vi "SP Execute Test.vi"(1 "CH Controls":T13[](array[typedef]) {"Measure" items=["S11", "S21", "S12", "S22"]; "Reference" format="%#.2g"; "Display Data" items=["Data", "Memory", "Data/Memory"]; "Format" items=["Log Mag", "Phase", "Expanded Phase", "Delay", "Smith", "Polar", "Lin Mag", "SWR", "Loss", "Real", "Imaginary"]; "Scale" min=0.001 step=1.0 format="%#.2g"; "Position" min=0.0 max=10.0}, 5 "Seq Count":u32, 7 "Timing Metrics In":string, 9 "Test Parameters":T20={"Stimulus"={"Use Instrument Settings"=FALSE, "Blank Frequencies"=FALSE, "Sweep Type"=enum."Linear", "Sweep"={"Fstart"=500.0, "Fstop"=1500.0, "Units"=enum."MHz", "Points"=2}, "Power (dBm)"=999.0, "IFBW (Hz)"=-1.0, "Sweep Time (s)"=-1.0, "Calibration"={"State"=FALSE, "String"=""}}, "Measurement"={"Auto Select"=TRUE, "Data Source"=enum."VNA", "Ports"=2, "Parameters"=[]}, "De-Embed"={"De-Embed"=FALSE, "Adapters"=[]}, "Display"={"Lock Control"=FALSE, "Retain Settings"=TRUE, "Formatted Data"=FALSE, "Plot Orientation"=enum."Single", "Plot Controls"=[{"Trace Orientation"=enum."Overlay", "Frequency"={"Change Frequency"=FALSE, "Start"=500.0, "Stop"=1500.0, "Units"=enum."MHz"}, "Markers"=[], "Traces"=[]}, {"Trace Orientation"=enum."Overlay", "Frequency"={"Change Frequency"=FALSE, "Start"=500.0, "Stop"=1500.0, "Units"=enum."MHz"}, "Markers"=[], "Traces"=[]}, {"Trace Orientation"=enum."Overlay", "Frequency"={"Change Frequency"=FALSE, "Start"=500.0, "Stop"=1500.0, "Units"=enum."MHz"}, "Markers"=[], "Traces"=[]}, {"Trace Orientation"=enum."Overlay", "Frequency"={"Change Frequency"=FALSE, "Start"=500.0, "Stop"=1500.0, "Units"=enum."MHz"}, "Markers"=[], "Traces"=[]}]}, "Limits"=[], "Filter Limits"=[]} {"Filter Limits"."Parameter"."Stimulus Port" min=1 step=1; "Filter Limits"."Parameter"."Response Port" min=1 step=1; "Filter Limits"."Passband"."Bandwidth Attn" format="%.3g"; "Filter Limits"."Passband"."Stop/Span" format="%.3g"; "Filter Limits"."Passband"."Start/Center" format="%.3g"; "Measurement"."Parameters"."Channel" min=0 max=32 step=1; "Measurement"."Parameters"."Parameter"."Stimulus Port" min=1 step=1; "Measurement"."Parameters"."Parameter"."Response Port" min=1 step=1; "Limits"."Parameter"."Stimulus Port" min=1 step=1; "Limits"."Parameter"."Response Port" min=1 step=1; "Stimulus"."Sweep Time (s)" format="%.3g"; "Display"."Plot Controls"."Traces"."Reference" format="%#.2g"; "Display"."Plot Controls"."Traces"."Display Data" items=["Data", "Memory", "Data/Memory"]; "Display"."Plot Controls"."Traces"."Format" items=["Log Mag", "Phase", "Expanded Phase", "Delay", "Smith", "Polar", "Lin Mag", "SWR", "Loss", "Real", "Imaginary"]; "Display"."Plot Controls"."Traces"."Scale" min=0.001 step=1.0 format="%#.2g"; "Display"."Plot Controls"."Traces"."Position" min=0.0 max=10.0; "Display"."Plot Controls"."Frequency"."Stop" format="%.3g"; "Display"."Plot Controls"."Frequency"."Start" format="%.3g"}, 11 "error in (no error)":errorcluster, 12 "Driver Refs":T16, 13 "Instrument Record":T9) -> (3 "Limit Results":T1[](array[typedef]) {"Parameter"."Stimulus Port" min=1 step=1; "Parameter"."Response Port" min=1 step=1}, 4 "Results":waveform(dbl)[](array[waveform]), 6 "Memory Exists?":bool[](array[boolean]), 8 "Timing Metrics Out":string, 10 "Parameters Measured":T10[](array[typedef]) {"Channel" min=1 max=99 step=1; "Parameter"."Stimulus Port" min=1 step=1; "Parameter"."Response Port" min=1 step=1}, 14 "Passed?":bool, 15 "error out":errorcluster)   [LabVIEW 2011]
uses:
  TypeDefs/SP Test Parameters.ctl
  TypeDefs/SP Stimulus Parameters.ctl
  TypeDefs/SP Frequency Units.ctl
  TypeDefs/SP Calibration State.ctl
  TypeDefs/SP Measurement.ctl
  TypeDefs/SP Parameters.ctl
  TypeDefs/SP Parameter.ctl
  TypeDefs/SP De-Embed.ctl
  TypeDefs/SP Adapter.ctl
  TypeDefs/SP Data.ctl
  TypeDefs/SP Display Parameters.ctl
  TypeDefs/SP Display Plot Controls Cluster.ctl
  TypeDefs/SP Marker Cluster.ctl
  TypeDefs/SP Marker Type.ctl
  TypeDefs/SP Display Trace Controls.ctl
  TypeDefs/SP Display Format.ctl
  TypeDefs/SP Display Data.ctl
  TypeDefs/SP Limit.ctl
  TypeDefs/SP Format.ctl
  TypeDefs/SP Limit Type.ctl
  TypeDefs/SP Limit Point.ctl
  Test Referential Limit.ctl
  TypeDefs/SP Filter.ctl
  TypeDefs/SP Filter Type.ctl
  TypeDefs/SP Filter Passband.ctl
  TypeDefs/SP Frequency Format.ctl
  TypeDefs/SP Filter Ripple.ctl
  TypeDefs/SP Attenuation Point.ctl
  TypeDefs/SP Attenuation Type.ctl
  TypeDefs/SP Skirt Rejection Point.ctl
  TypeDefs/SP Relative Loss.ctl
  TypeDefs/SP Driver Refs.ctl
  drivers/VNA/VNA Driver Ref.ctl
  drivers/SNA/SNA Driver Ref.ctl
  drivers/IMP/IMP Driver Ref.ctl
  TypeDefs/SP Parameter to Measure.ctl
  TypeDefs/SP Measurement Format.ctl
  typedefs/Instrument Record.ctl
  TypeDefs/SP Limit Results.ctl
  TypeDefs/SP Bandwidth Limit Results.ctl
  TypeDefs/SP Ripple Limit Results.ctl
  TypeDefs/SP Attenuation Limit Results.ctl
  TypeDefs/SP Skirt Limit Results.ctl
  TypeDefs/SP Miscellaneous Parameters.ctl
  drivers/VNA/VNA Command.ctl
  drivers/SNA/SNA Command.ctl
  drivers/IMP/S2P/TypeDefs/S2P IMP Measurement Data.ctl
  drivers/IMP/IMP Command.ctl
panel:
  in  "Empty Results":waveform(dbl)[](array[waveform])
  # "Div"
  # "Div"
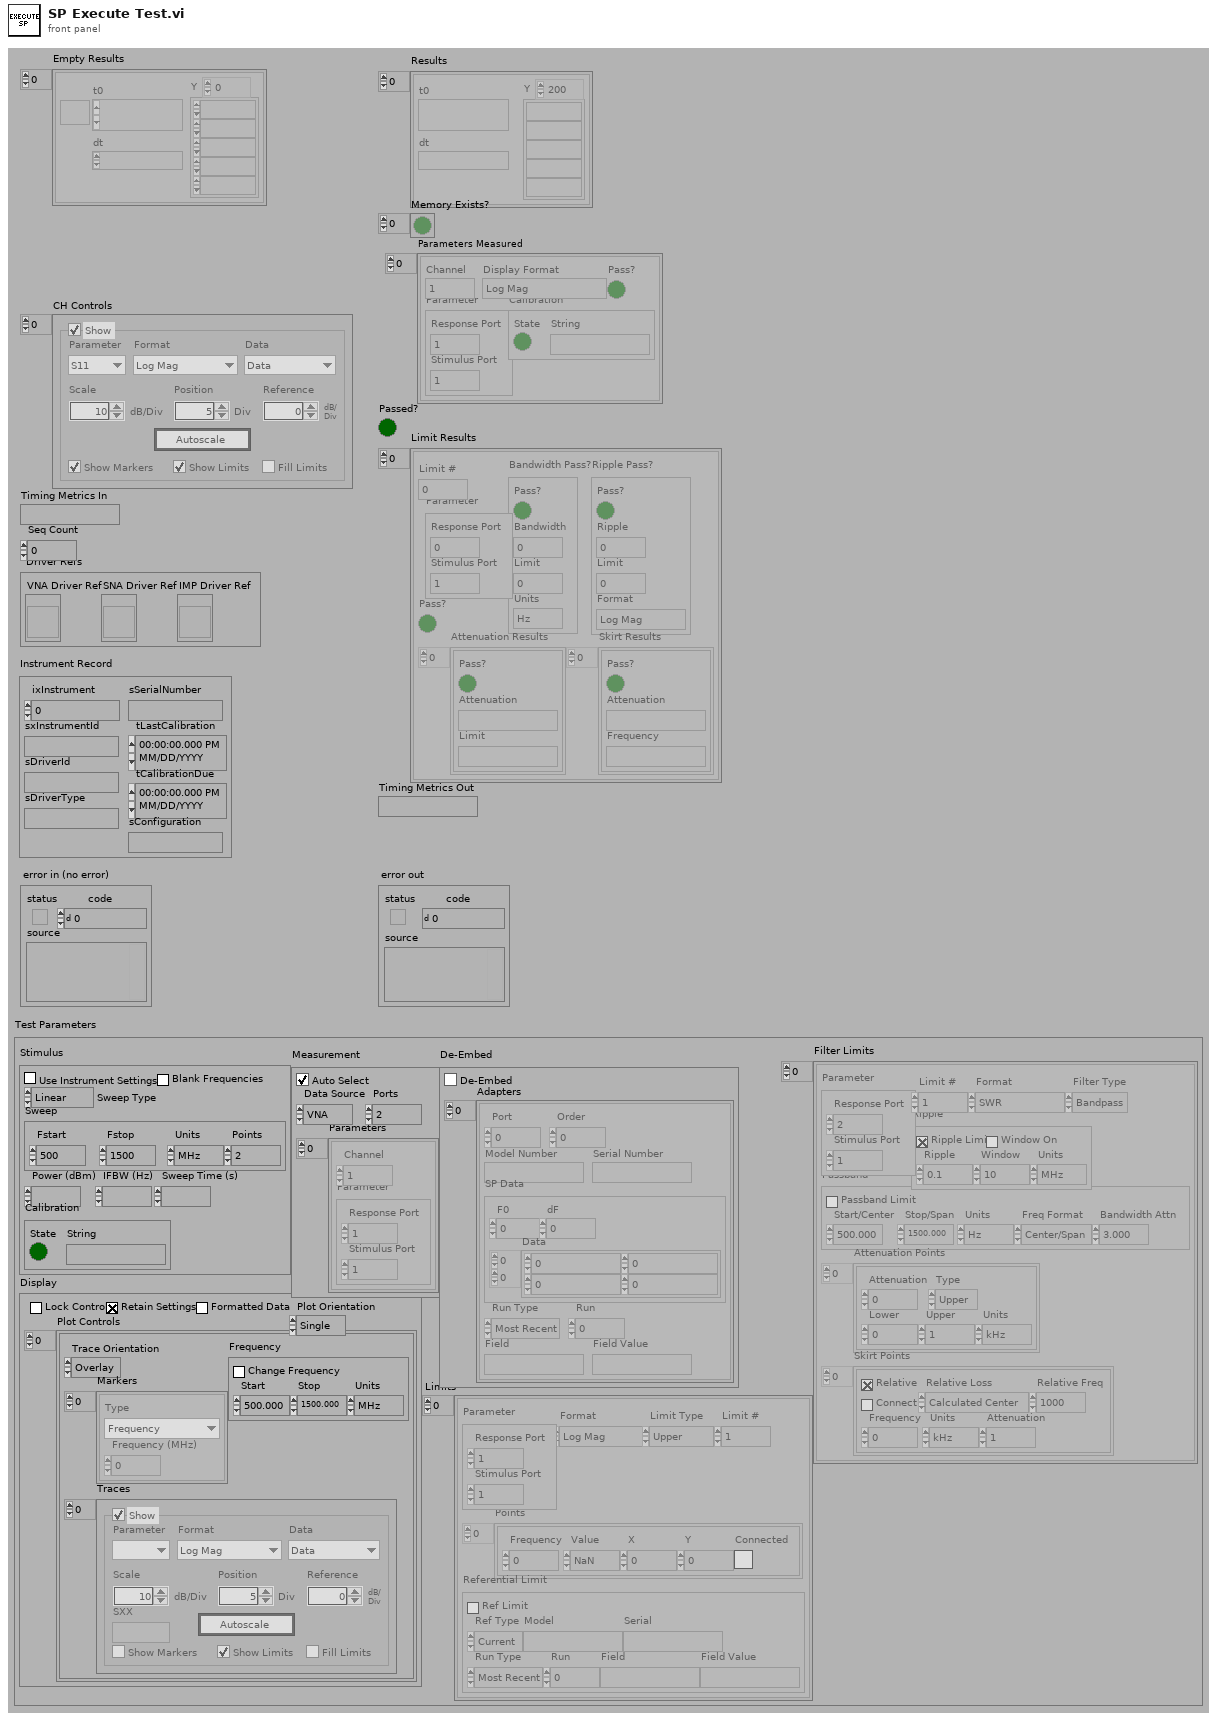
[diagram p1: front panel]
types:
  T1 = typedef "SP Limit Results.ctl" = cluster{"Limit #":i8, "Parameter":T2, "Bandwidth Pass?":T3, "Ripple Pass?":T5, "Attenuation Results":T7[], "Skirt Results":T8[], "Pass?":bool}
  T2 = typedef "SP Parameter.ctl" = cluster{"Stimulus Port":i8, "Response Port":i8}
  T3 = typedef "SP Bandwidth Limit Results.ctl" = cluster{"Pass?":bool, "Bandwidth":dbl, "Limit":dbl, "Units":T4}
  T4 = typedef "SP Frequency Units.ctl" = enum16{"Hz", "kHz", "MHz", "GHz", "Points"}
  T5 = typedef "SP Ripple Limit Results.ctl" = cluster{"Pass?":bool, "Ripple":dbl, "Limit":dbl, "Format":T6}
  T6 = typedef "SP Format.ctl" = enum16{"Log Mag", "Lin Mag", "SWR", "Phase", "Expanded Phase", "Delay", "Insertion Loss", "Isolation", "Return Loss"}
  T7 = typedef "SP Attenuation Limit Results.ctl" = cluster{"Pass?":bool, "Attenuation":string, "Limit":string}
  T8 = typedef "SP Skirt Limit Results.ctl" = cluster{"Pass?":bool, "Attenuation":string, "Frequency":string}
  T9 = typedef "Instrument Record.ctl" = cluster{"ixInstrument":i32, "sxInstrumentId":string, "sDriverId":string, "sDriverType":string, "sSerialNumber":string, "tLastCalibration":timestamp, "tCalibrationDue":timestamp, "sConfiguration":string}
  T10 = typedef "SP Parameter to Measure.ctl" = cluster{"Channel":i8, "Parameter":T2, "Calibration":T11, "Display Format":T12, "Pass?":bool}
  T11 = typedef "SP Calibration State.ctl" = cluster{"State":bool, "String":string}
  T12 = typedef "SP Measurement Format.ctl" = enum32{"Log Mag", "Phase", "Delay", "Smith (R+jX)", "Polar (Re/Im)", "Linear Mag", "SWR", "Real", "Imaginary", "Smith (Lin/Phase)", "Smith (Log/Phase)", "Smith (Real/Imag)", "Smith (G+jB)", "Polar (Lin/Phase)", "Polar (Log/Phase)", "Expanded Phase", "Positive Phase", "Inverted Smith", "Unwrapped Phase", "Power Out", "Power In", "Linear Mag/Phase", "Log Mag/Phase", "Real/Imaginary"}
  T13 = typedef "SP Display Trace Controls.ctl" = cluster{"Trace On":bool, "Measure":i32, "Format":T14, "Autoscale":bool, "Reference":dbl, "\nRefUnit":string, "Position":dbl, "Scale":dbl, "ScaleUnit":string, "LimitOn":bool, "LimitFill":bool, "Display Data":T15, "Show Markers":bool, "SXX":string}
  T14 = typedef "SP Display Format.ctl" = i32
  T15 = typedef "SP Display Data.ctl" = u16
  T16 = typedef "SP Driver Refs.ctl" = cluster{"VNA Driver Ref":T17, "SNA Driver Ref":T18, "IMP Driver Ref":T19}
  T17 = typedef "VNA Driver Ref.ctl" = refnum<vi>
  T18 = typedef "SNA Driver Ref.ctl" = refnum<vi>
  T19 = typedef "IMP Driver Ref.ctl" = refnum<vi>
  T20 = typedef "SP Test Parameters.ctl" = cluster{"Stimulus":T21, "Measurement":T22, "De-Embed":T24, "Display":T27, "Limits":T31[], "Filter Limits":T35[]}
  T21 = typedef "SP Stimulus Parameters.ctl" = cluster{"Use Instrument Settings":bool, "Blank Frequencies":bool, "Sweep Type":enum32{"Linear", "Logarithmic", "List", "Power", "CW"}, "Sweep":cluster{"Fstart":dbl, "Fstop":dbl, "Units":T4, "Points":i32}, "Power (dBm)":dbl, "IFBW (Hz)":dbl, "Sweep Time (s)":dbl, "Calibration":T11}
  T22 = typedef "SP Measurement.ctl" = cluster{"Auto Select":bool, "Data Source":enum16{"VNA", "Data File"}, "Ports":i8, "Parameters":T23[]}
  T23 = typedef "SP Parameters.ctl" = cluster{"Channel":i8, "Parameter":T2}
  T24 = typedef "SP De-Embed.ctl" = cluster{"De-Embed":bool, "Adapters":T25[]}
  T25 = typedef "SP Adapter.ctl" = cluster{"Port":i8, "Order":i8, "Model Number":string, "Serial Number":string, "SP Data":T26, "Run Type":enum16{"Most Recent", "Run #", "Match Field"}, "Run":i32, "Field":string, "Field Value":string}
  T26 = typedef "SP Data.ctl" = cluster{"F0":dbl, "dF":dbl, "Data":cdb[][]}
  T27 = typedef "SP Display Parameters.ctl" = cluster{"Lock Control":bool, "Retain Settings":bool, "Formatted Data":bool, "Plot Orientation":enum32{"Single", "Dual", "Quad"}, "Plot Controls":T28[]}
  T28 = typedef "SP Display Plot Controls Cluster.ctl" = cluster{"Trace Orientation":enum32{"Overlay", "Split"}, "Frequency":cluster{"Change Frequency":bool, "Start":dbl, "Stop":dbl, "Units":T4}, "Markers":T29[], "Traces":T13[]}
  T29 = typedef "SP Marker Cluster.ctl" = cluster{"Type":T30, "Frequency (MHz)":dbl}
  T30 = typedef "SP Marker Type.ctl" = enum16{"Frequency", "Trace Maximum", "Trace Minimum", "Limit Maximum", "Limit Minimum"}
  T31 = typedef "SP Limit.ctl" = cluster{"Parameter":T2, "Format":T6, "Limit Type":T32, "Points":T33[], "Referential Limit":T34, "Limit #":i8}
  T32 = typedef "SP Limit Type.ctl" = enum16{"Upper", "Lower", "Delta", "Filter", "Referential"}
  T33 = typedef "SP Limit Point.ctl" = cluster{"Frequency":dbl, "Value":dbl, "X":dbl, "Y":dbl, "Connected":bool}
  T34 = typedef "Test Referential Limit.ctl" = cluster{"Ref Limit":bool, "Ref Type":enum16{"Current", "Specify"}, "Model":string, "Serial":string, "Run Type":enum16{"Most Recent", "Run #", "Match Field"}, "Run":i32, "Field":string, "Field Value":string}
  T35 = typedef "SP Filter.ctl" = cluster{"Limit #":i8, "Parameter":T2, "Format":T6, "Filter Type":T36, "Passband":T37, "Ripple":T39, "Attenuation Points":T40[], "Skirt Points":T42[]}
  T36 = typedef "SP Filter Type.ctl" = enum16{"Lowpass", "Highpass", "Bandpass", "Bandstop"}
  T37 = typedef "SP Filter Passband.ctl" = cluster{"Start/Center":dbl, "Stop/Span":dbl, "Units":T4, "Freq Format":T38, "Bandwidth Attn":dbl, "Passband Limit":bool}
  T38 = typedef "SP Frequency Format.ctl" = enum16{"Start/Stop", "Center/Span"}
  T39 = typedef "SP Filter Ripple.ctl" = cluster{"Ripple Limit":bool, "Window On":bool, "Ripple":dbl, "Window":dbl, "Units":T4}
  T40 = typedef "SP Attenuation Point.ctl" = cluster{"Attenuation":dbl, "Type":T41, "Lower":dbl, "Upper":dbl, "Units":T4}
  T41 = typedef "SP Attenuation Type.ctl" = enum16{"Center", "Lower", "Upper"}
  T42 = typedef "SP Skirt Rejection Point.ctl" = cluster{"Relative":bool, "Connect":bool, "Frequency":dbl, "Units":T4, "Attenuation":dbl, "Relative Loss":T43, "Relative Freq":dbl}
  T43 = typedef "SP Relative Loss.ctl" = enum16{"Calculated Center", "Passband Minimum", "Passband Maximum", "Passband Average", "Frequency"}
  T44 = cluster{"Measurement Units":T4, "Display Units":T4}
  T45 = typedef "SP Miscellaneous Parameters.ctl" = cluster{"Formatted Data":bool, "Auto Select":bool, "Seq Count":u32}
  T46 = typedef "VNA Command.ctl" = enum16{"LOAD", "INITIALIZE", "PRESET", "GET STIMULUS", "SET STIMULUS", "GET CALIBRATION", "CALIBRATE", "RESTORE", "MEASURE", "RELEASE", "UNLOAD", "CONFIRM", "SORT"}
  T47 = typedef "SNA Command.ctl" = enum16{"LOAD", "INITIALIZE", "PRESET", "GET STIMULUS", "SET STIMULUS", "GET CALIBRATION", "CALIBRATE", "RESTORE", "MEASURE", "RELEASE", "UNLOAD", "CONFIRM", "SORT"}
  T48 = typedef "S2P IMP Measurement Data.ctl" = cluster{"Parameters Measured":T10[], "S2P Data":T26}
  T49 = typedef "IMP Command.ctl" = enum16{"LOAD", "INITIALIZE", "IMPORT", "UNLOAD"}
  T50 = cluster{"F0":dbl, "dF":dbl, "Formatted Values":dbl[]}
  T51 = cluster{"Bandwidth Attn":dbl, "Center Freq (MHz)":dbl, "Span Freq (MHz)":dbl, "Pass?":bool, "Bandwidth (MHz)":dbl, "Bandwidth Limit (MHz)":dbl, "Attenuation Points":dbl[]}
  T52 = cluster{"Upper Limit":cluster{"F0":dbl, "dF":dbl, "Formatted Values":dbl[]}, "Lower Limit":cluster{"F0":dbl, "dF":dbl, "Formatted Values":dbl[]}}
  T53 = cluster{"UPass?":bool, "LPass?":bool, "Frequency":dbl, "Lower Limit":dbl, "Upper Limit":dbl, "Type":T41}[]
  T54 = cluster{"x0":dbl, "dx":dbl, "Stored Values":dbl[]}
  T55 = cluster{cluster{"x0":dbl, "dx":dbl, "Stored Values":dbl[]}, cluster{"x0":dbl, "dx":dbl, "Stored Values":dbl[]}}
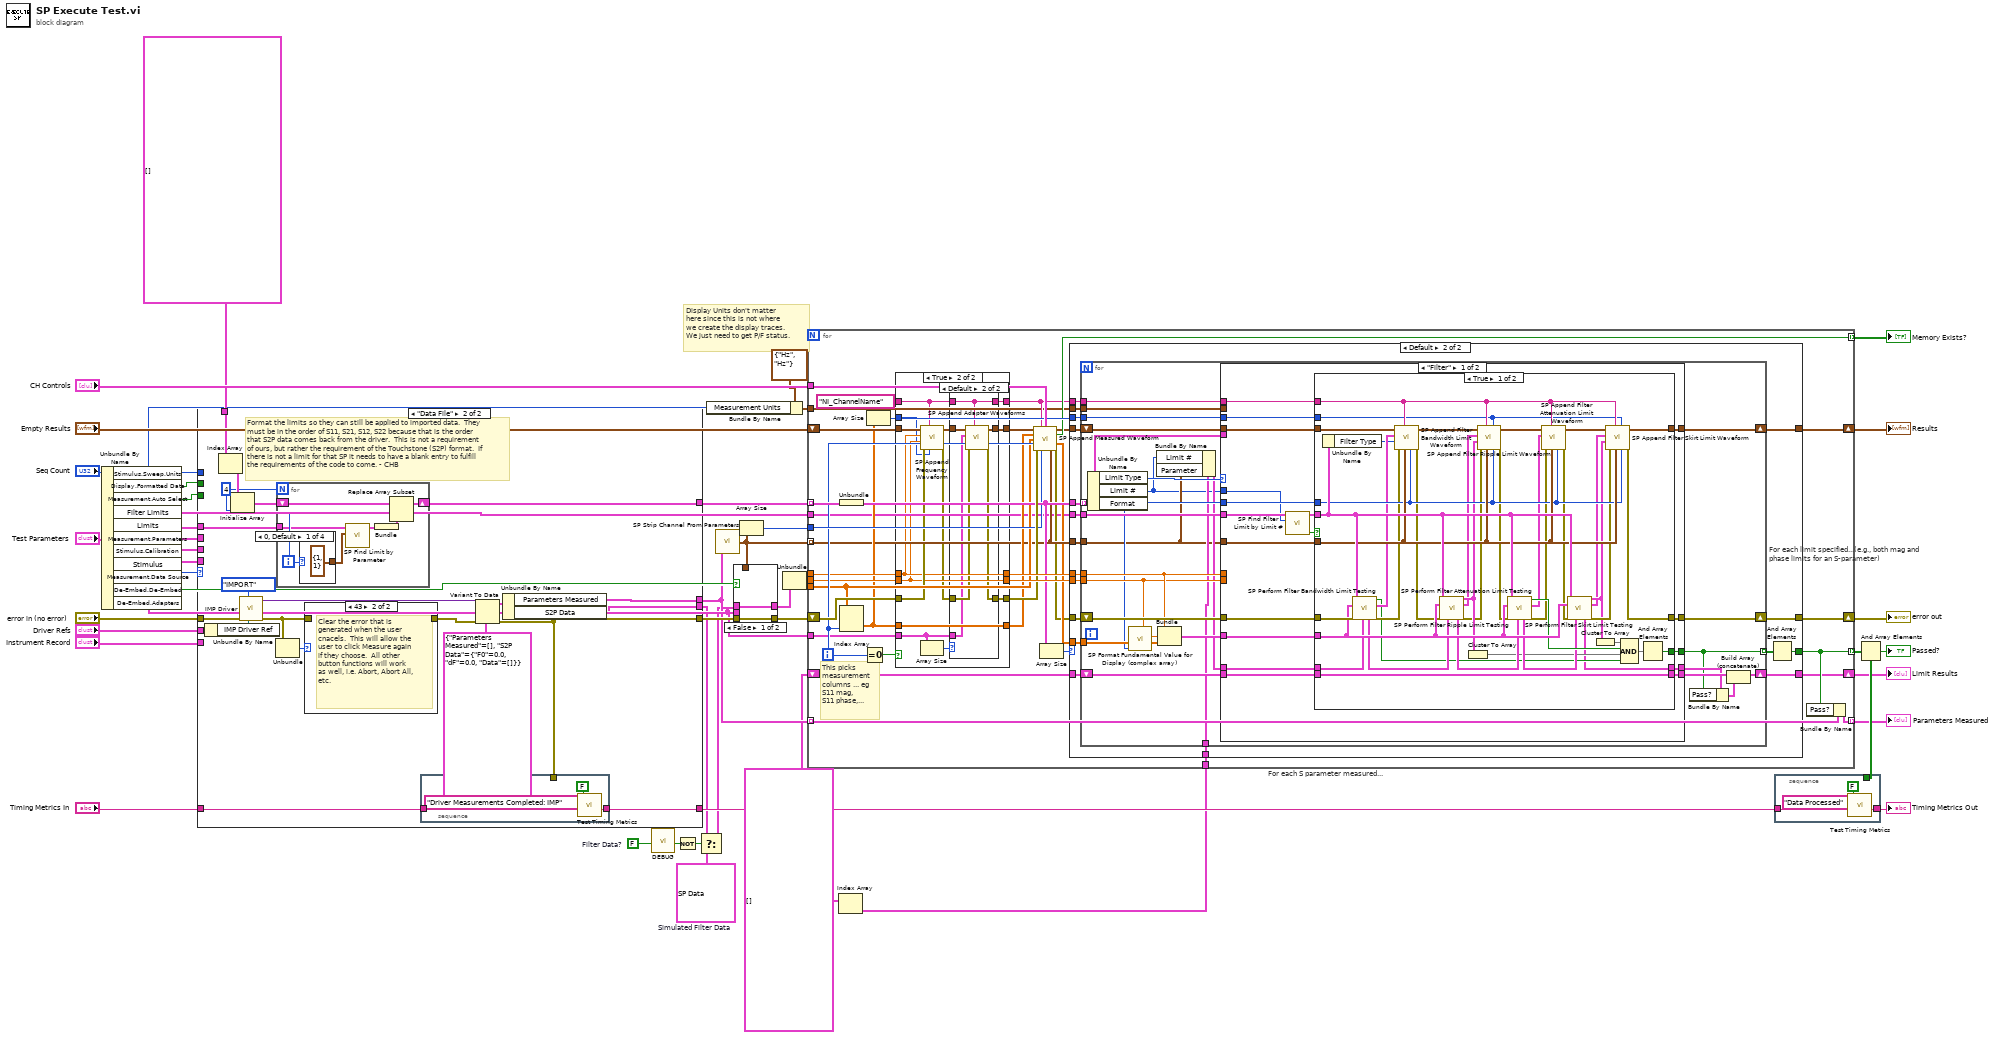
[diagram p0: block diagram]
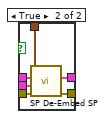
[diagram p2: hidden frame]
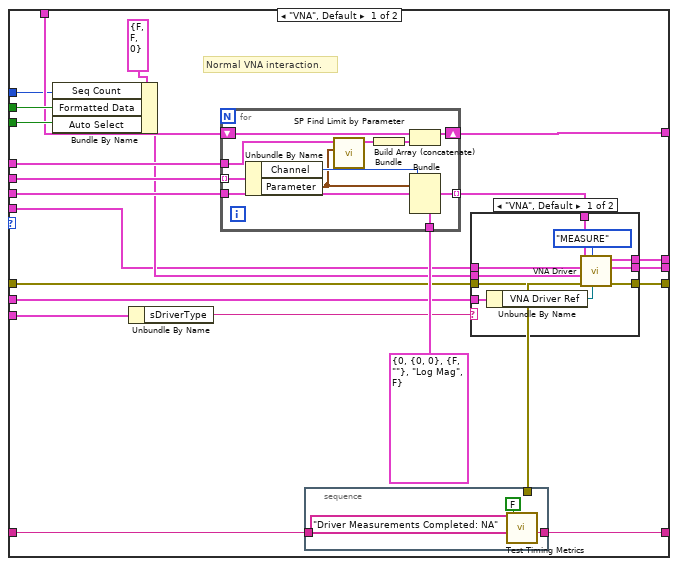
[diagram p3: hidden frame]
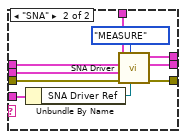
[diagram p4: hidden frame]
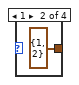
[diagram p6: hidden frame]
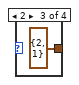
[diagram p7: hidden frame]
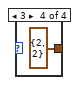
[diagram p8: hidden frame]
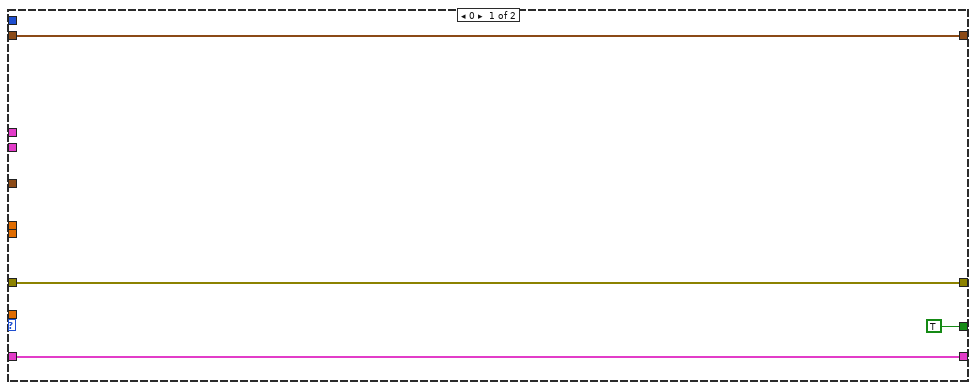
[diagram p9: hidden frame]
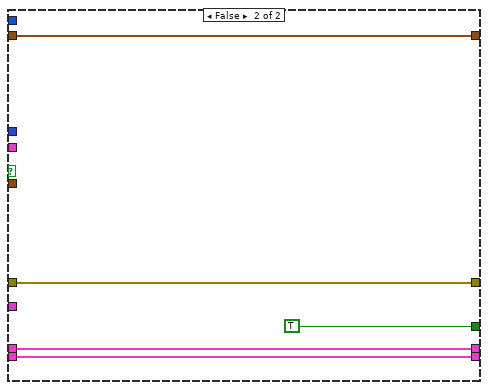
[diagram p10: hidden frame]
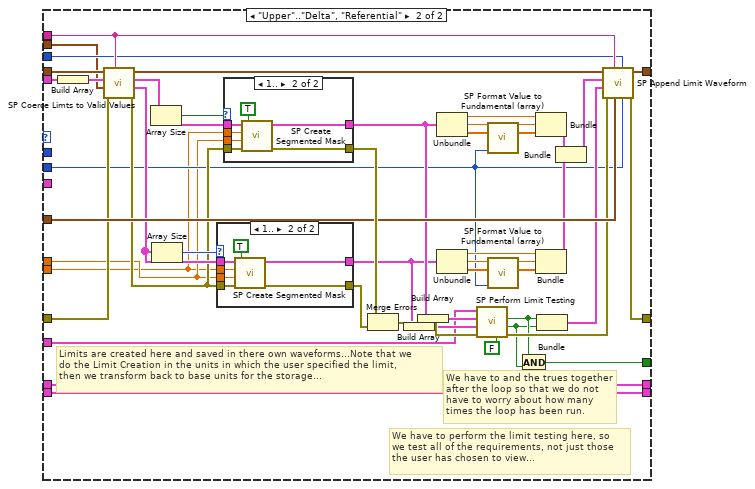
[diagram p11: hidden frame]
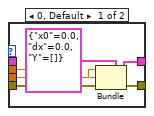
[diagram p12: hidden frame]
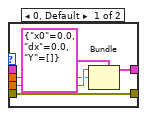
[diagram p13: hidden frame]
diagram:
  w3 = T1[] []
  w9 = FALSE  # Filter Data?
  w6 = T26 {"F0"=1700.0, "dF"=1.0, "Data"=[[-0.6018883288138366-0.2912013889246391i, 0.25843199895687796+0.6001894532665946i, 1.0+0.0i, 1.0+0.0i], [-0.5763938433657362-0.16773283578975615i, 0.37772558398449546+0.6071698116448432i, 1.0+0.0i, 1.0+0.0i], [-0.519689947876343-0.05406961123928598i, 0.5054119893123452+0.5838015468749106i, 1.0+0.0i, 1.0+0.0i], [-0.4366631932536643+0.038653140967053336i, 0.6323001346464633+0.5273763672849814i, 1.0+0.0i, 1.0+0.0i], [-0.3367762107137387+0.10167424321959725i, 0.7461057345374577+0.4390505932852546i, 1.0+0.0i, 1.0+0.0i], [-0.23206146469338626+0.1317558747901435i, 0.8374292632292502+0.3249695878798761i, 1.0+0.0i, 1.0+0.0i], [-0.13428970687981837+0.1316706711180515i, 0.900317905750139+0.1948071131291862i, 1.0+0.0i, 1.0+0.0i], [-0.0519954009317567+0.10798684987828776i, 0.9338709717280576+0.05829020485907047i, 1.0+0.0i, 1.0+0.0i], [0.010578915376855002+0.06919151060092682i, 0.9411153215780537-0.07694445704762284i, 1.0+0.0i, 1.0+0.0i], [0.05258172168640398+0.02288386508379801i, 0.9247525186312551-0.20416450691947172i, 1.0+0.0i, 1.0+0.0i], [0.07586320408971295-0.02427093912251751i, 0.8912400676746711-0.3217436008032638i, 1.0+0.0i, 1.0+0.0i], [0.0834246197482034-0.06790328480338377i, 0.8439917666780876-0.42831686461220936i, 1.0+0.0i, 1.0+0.0i], [0.07866808071336005-0.10505806260292615i, 0.78641056187367-0.5234791187831817i, 1.0+0.0i, 1.0+0.0i], [0.06489162284893765-0.13445634684056035i, 0.7212501289028754-0.6083145624168425i, 1.0+0.0i, 1.0+0.0i], [0.04507227165494071-0.15522420928026068i, 0.6495134688280773-0.6824883986293371i, 1.0+0.0i, 1.0+0.0i], [0.02186237509833218-0.16744628811960777i, 0.5727083373218407-0.7463211066382691i, 1.0+0.0i, 1.0+0.0i], [-0.0028246619373131676-0.17163375094123137i, 0.4918939724054302-0.8016715915329948i, 1.0+0.0i, 1.0+0.0i], [-0.02714462258660534-0.16846044251443718i, 0.40771953951852236-0.848048518977557i, 1.0+0.0i, 1.0+0.0i], [-0.04965487991424324-0.15891144281898575i, 0.32087934927959744-0.8851169409466159i, 1.0+0.0i, 1.0+0.0i], [-0.06940115989214148-0.14395347580736373i, 0.23105911621068337-0.9151527346496748i, 1.0+0.0i, 1.0+0.0i], [-0.08515954507306635-0.12468116376469908i, 0.1403489417912114-0.9346160952374049i, 1.0+0.0i, 1.0+0.0i], [-0.09674321476559439-0.1023120232228757i, 0.04818766902243024-0.9456399069017796i, 1.0+0.0i, 1.0+0.0i], [-0.10384848778239429-0.07792886127276757i, -0.044093597115198176-0.9476633622454788i, 1.0+0.0i, 1.0+0.0i], [-0.10642398257790069-0.052629906048574614i, -0.13557150924760691-0.9402477642662153i, 1.0+0.0i, 1.0+0.0i], [-0.10447933019033262-0.027496582837167702i, -0.22651251036758296-0.9249390180549153i, 1.0+0.0i, 1.0+0.0i], [-0.09846522597296979-0.0033023854612930694i, -0.3150646229058073-0.9007516295430944i, 1.0+0.0i, 1.0+0.0i], [-0.08867113842250143+0.018985327208484115i, -0.3996975613559442-0.867381307278978i, 1.0+0.0i, 1.0+0.0i], [-0.07586177040152732+0.03886020162270151i, -0.4809323563603943-0.8261918442002553i, 1.0+0.0i, 1.0+0.0i], [-0.06076646059838993+0.055993218767238i, -0.5581660126308761-0.7778153443708942i, 1.0+0.0i, 1.0+0.0i], [-0.04381207606238176+0.06982104609066907i, -0.6287295195292726-0.7219563939864023i, 1.0+0.0i, 1.0+0.0i], [-0.02591401637984273+0.08040210957536097i, -0.6940277277339839-0.6599926809567306i, 1.0+0.0i, 1.0+0.0i], [-0.007662933312265582+0.08775248303207699i, -0.7520150911557977-0.5921261482908812i, 1.0+0.0i, 1.0+0.0i], [0.010327353173893283+0.09204591847645842i, -0.8054632379209045-0.5195334217200286i, 1.0+0.0i, 1.0+0.0i], [0.027570187893991904+0.09328646897248352i, -0.8495372541500987-0.4423692583583411i, 1.0+0.0i, 1.0+0.0i], [0.043636518509812976+0.09203190924415088i, -0.8866024628267639-0.3616497030468273i, 1.0+0.0i, 1.0+0.0i], [0.05815857292883628+0.08853217374133557i, -0.916102803615982-0.2779561134304512i, 1.0+0.0i, 1.0+0.0i], [0.07092777290362523+0.08316021939919031i, -0.9371691434087805-0.19228967425838717i, 1.0+0.0i, 1.0+0.0i], [0.08166451250945678+0.07633417924416686i, -0.9513886911911866-0.10464605910605339i, 1.0+0.0i, 1.0+0.0i], [0.09032871637381922+0.06840197558392054i, -0.956826030767709-0.016280501409187128i, 1.0+0.0i, 1.0+0.0i], [0.09705657838026943+0.05972833435455881i, -0.9541463163875222+0.07225510514550987i, 1.0+0.0i, 1.0+0.0i], [0.1017157657878945+0.05065605850842947i, -0.9433210671957775+0.16034009806172234i, 1.0+0.0i, 1.0+0.0i], [0.10448012976900736+0.041427625084476484i, -0.9245071206581749+0.2471693341448325i, 1.0+0.0i, 1.0+0.0i], [0.10542608402879289+0.032428786673877275i, -0.8975198220345031+0.33217007008156507i, 1.0+0.0i, 1.0+0.0i], [0.10466470261736624+0.02365108018246849i, -0.8626567303162795+0.414682914555206i, 1.0+0.0i, 1.0+0.0i], [0.10230330280167362+0.015328926437470256i, -0.8200935976978028+0.4940875957110222i, 1.0+0.0i, 1.0+0.0i], [0.09860433016372575+0.007612820033679798i, -0.7699420524716706+0.5693633026244502i, 1.0+0.0i, 1.0+0.0i], [0.09368580974287007+0.0005573491927782479i, -0.7125436571337076+0.6399868897098582i, 1.0+0.0i, 1.0+0.0i], [0.08756119563288138-0.005806518604850663i, -0.6484962392852844+0.7060130026305704i, 1.0+0.0i, 1.0+0.0i], [0.08041985909062076-0.011148728567773908i, -0.5775952397661317+0.7645606455570968i, 1.0+0.0i, 1.0+0.0i], [0.0721923675580467-0.01580110179377119i, -0.5008883448891464+0.8164731956480251i, 1.0+0.0i, 1.0+0.0i], [0.06304326080671951-0.019419514076621566i, -0.41869765614671717+0.8622852805854512i, 1.0+0.0i, 1.0+0.0i], [0.053113941666137324-0.02208180740934336i, -0.3318925693769244+0.8993924639844907i, 1.0+0.0i, 1.0+0.0i], [0.042327853302586-0.023652514838652564i, -0.24055892940082874+0.9288413877153515i, 1.0+0.0i, 1.0+0.0i], [0.030838926552563258-0.02377923837039422i, -0.1461630870200274+0.94816630091127i, 1.0+0.0i, 1.0+0.0i], [0.01870982273255544-0.02249094220644248i, -0.04987288285879495+0.9566115126117133i, 1.0+0.0i, 1.0+0.0i], [0.006143225202847295-0.019632915523019934i, 0.04882759736918653+0.9571527194865719i, 1.0+0.0i, 1.0+0.0i], [-0.006649233662454022-0.014947621089703395i, 0.14785104513947628+0.9464339527379307i, 1.0+0.0i, 1.0+0.0i], [-0.01940066611782043-0.008320788091237083i, 0.24621363044144073+0.9252244724465958i, 1.0+0.0i, 1.0+0.0i], [-0.031724477990716045+0.0004593234166332625i, 0.34334164002308953+0.8934780479138885i, 1.0+0.0i, 1.0+0.0i], [-0.04314760762766865+0.011362796606390155i, 0.4358039550543813+0.8497553136816223i, 1.0+0.0i, 1.0+0.0i], [-0.05318862373029016+0.024395123071694384i, 0.5259021789709166+0.7966200883485474i, 1.0+0.0i, 1.0+0.0i], [-0.06127106944236175+0.03943945567223453i, 0.6097426634187605+0.7326566320758651i, 1.0+0.0i, 1.0+0.0i], [-0.06679234071688708+0.05615716369606713i, 0.6867663672489616+0.6586197824203649i, 1.0+0.0i, 1.0+0.0i], [-0.0691744018739379+0.07405494542895746i, 0.7564985991167886+0.575499578950503i, 1.0+0.0i, 1.0+0.0i], [-0.06791698397038357+0.09252578356037992i, 0.8155353867263107+0.48347895828640297i, 1.0+0.0i, 1.0+0.0i], [-0.06252754216094453+0.11062154548610267i, 0.8642232625000523+0.3839108643796431i, 1.0+0.0i, 1.0+0.0i], [-0.05288141014773409+0.12739587954612072i, 0.9028158825599887+0.2775523651413829i, 1.0+0.0i, 1.0+0.0i], [-0.03894579332671778+0.14139470266136236i, 0.9280152441914633+0.16565062882775497i, 1.0+0.0i, 1.0+0.0i], [-0.021125341496806904+0.151477317248256i, 0.939894734553657+0.04956449848513996i, 1.0+0.0i, 1.0+0.0i], [-8.54153469215474e-05+0.15640582926585647i, 0.9376456681984923-0.06977512732062516i, 1.0+0.0i, 1.0+0.0i], [0.022929291642011577+0.15463846381715032i, 0.9199704468055506-0.19057784118682192i, 1.0+0.0i, 1.0+0.0i], [0.0464693495485323+0.14532227623577607i, 0.8863437141821184-0.31187044472783965i, 1.0+0.0i, 1.0+0.0i], [0.06796233423343687+0.12734375811660376i, 0.8345695367569668-0.4302649312109253i, 1.0+0.0i, 1.0+0.0i], [0.08500727751830782+0.10086621442731726i, 0.7647210645029121-0.5439587069427498i, 1.0+0.0i, 1.0+0.0i], [0.09449733566311004+0.06653208034100902i, 0.6762524317082488-0.6516719436743442i, 1.0+0.0i, 1.0+0.0i], [0.09329074668210832+0.026321785808147646i, 0.5677674949875572-0.7475681327174338i, 1.0+0.0i, 1.0+0.0i], [0.07865411994723565-0.016508336787470018i, 0.4400858149871239-0.8284769003283825i, 1.0+0.0i, 1.0+0.0i], [0.048803583668660194-0.0568001919793608i, 0.29465269320802007-0.8871734175171272i, 1.0+0.0i, 1.0+0.0i], [0.004182352171136945-0.08856370429529446i, 0.13510538282317108-0.9200123504592056i, 1.0+0.0i, 1.0+0.0i], [-0.05189515517396443-0.10516354963437015i, -0.03461173094638121-0.9233734570999651i, 1.0+0.0i, 1.0+0.0i], [-0.11271195420288169-0.10107101325115063i, -0.20690768709244398-0.8922502814371098i, 1.0+0.0i, 1.0+0.0i], [-0.16829804569833243-0.07347514401271295i, -0.3761310850654713-0.8257529634002132i, 1.0+0.0i, 1.0+0.0i], [-0.20548548055427257-0.024164447740455296i, -0.5338367606432877-0.7225856659800891i, 1.0+0.0i, 1.0+0.0i], [-0.21060051222683637+0.03808315595329911i, -0.6754503727190233-0.582206612212459i, 1.0+0.0i, 1.0+0.0i], [-0.17032472418299607+0.094645061065754i, -0.7947447285843722-0.3996471781744263i, 1.0+0.0i, 1.0+0.0i], [-0.07901238526411039+0.11140467318220737i, -0.8731045878321936-0.16488328715630465i, 1.0+0.0i, 1.0+0.0i], [0.041070055012981034+0.03384566989630328i, -0.8699933934683103+0.12689815077259753i, 1.0+0.0i, 1.0+0.0i], [0.09522272596441572-0.18030821997863317i, -0.7129285845384136+0.4292365673144433i, 1.0+0.0i, 1.0+0.0i], [-0.057767881783225034-0.44141158140544073i, -0.3949063232879774+0.5979367576916298i, 1.0+0.0i, 1.0+0.0i], [-0.38286646504616595-0.5339233635346229i, -0.08370031841862433+0.5428128260911925i, 1.0+0.0i, 1.0+0.0i], [-0.6707547787277324-0.419775731598612i, 0.07825384819214672+0.37890749400285856i, 1.0+0.0i, 1.0+0.0i], [-0.8355857960356216-0.22314755441846254i, 0.12261040144112519+0.2345446292020144i, 1.0+0.0i, 1.0+0.0i], [-0.9037567438213129-0.028112762066985517i, 0.11602268884490194+0.1383535085737117i, 1.0+0.0i, 1.0+0.0i], [-0.9169998461744372+0.13988503290590304i, 0.0949845629822241+0.08011970193404727i, 1.0+0.0i, 1.0+0.0i], [-0.899930373556771+0.27988017559060463i, 0.07315580096005365+0.045728264987258994i, 1.0+0.0i, 1.0+0.0i], [-0.8661043528407536+0.39413340338314434i, 0.054553862622702655+0.025635892912699222i, 1.0+0.0i, 1.0+0.0i], [-0.8243936793307876+0.48912918769055636i, 0.03991819386209603+0.013977392878197612i, 1.0+0.0i, 1.0+0.0i], [-0.7784470995137205+0.5678115679587512i, 0.028825584139034185+0.0072632962697511015i, 1.0+0.0i, 1.0+0.0i], [-0.7313802800212125+0.6348899971679764i, 0.0205487395382581+0.003472387393030255i, 1.0+0.0i, 1.0+0.0i], [-0.6837688567671468+0.6918431623911119i, 0.014419840627457749+0.0014134892277889925i, 1.0+0.0i, 1.0+0.0i], [-0.6365134789438374+0.7389840725178888i, 0.009920944480821309+0.0003505747060961784i, 1.0+0.0i, 1.0+0.0i], [-0.5904763409864403+0.7796262634874056i, 0.006653837313751247-0.00011408053981226363i, 1.0+0.0i, 1.0+0.0i], [-0.5458038211957541+0.8138547282240669i, 0.004300523219497427-0.0002554306678072595i, 1.0+0.0i, 1.0+0.0i], [-0.5022644767687758+0.8443413526481423i, 0.0026253146522399397-0.00022918787711075504i, 1.0+0.0i, 1.0+0.0i], [-0.46063758969998697+0.870834484803912i, 0.001436091657660389-0.00012640370942258324i, 1.0+0.0i, 1.0+0.0i], [-0.4205212715176568+0.892056364965568i, 0.0006149818521453536+8.922068080420638e-06i, 1.0+0.0i, 1.0+0.0i], [-0.38157455147732555+0.9109817304805171i, 5.375518211271426e-05+0.00014240657180357867i, 1.0+0.0i, 1.0+0.0i], [-0.34485224565543604+0.9272549765683717i, -0.00030340377232163763+0.0002531608231524423i, 1.0+0.0i, 1.0+0.0i], [-0.309191519645884+0.9410922014349631i, -0.0005289154873562566+0.00034528784815929107i, 1.0+0.0i, 1.0+0.0i], [-0.27508884312629384+0.9529178397253227i, -0.0006338801843677425+0.00040466816161339894i, 1.0+0.0i, 1.0+0.0i], [-0.2422478680394226+0.9628926910109905i, -0.0006939871891300646+0.0004435554302594064i, 1.0+0.0i, 1.0+0.0i], [-0.21065570740800724+0.9713087070604108i, -0.0006949515854707573+0.00046688773728251464i, 1.0+0.0i, 1.0+0.0i], [-0.18035111079641905+0.9790944797425006i, -0.0006601754880812151+0.0004626549083955471i, 1.0+0.0i, 1.0+0.0i], [-0.15169164023575432+0.9843406039366385i, -0.0006093961095685952+0.0004535171636329728i, 1.0+0.0i, 1.0+0.0i], [-0.12372146793299463+0.9890405004689183i, -0.0005414837854990509+0.0004127167055461758i, 1.0+0.0i, 1.0+0.0i], [-0.09768245673341534+0.992354807438694i, -0.00047695038839787676+0.000376764639465228i, 1.0+0.0i, 1.0+0.0i], [-0.07113158541444688+0.9955308991485885i, -0.0004038033811464111+0.0003282452010286005i, 1.0+0.0i, 1.0+0.0i], [-0.04617189233186482+0.9984217287640034i, -0.0003280045495189821+0.0002832338432393144i, 1.0+0.0i, 1.0+0.0i], [-0.022718715629611558+0.9993491168638301i, -0.0002576920416455954+0.00022080872682340007i, 1.0+0.0i, 1.0+0.0i], [9.899373129130176e-05+1.0003391503941879i, -0.00018868362455628517+0.0001505864199428088i, 1.0+0.0i, 1.0+0.0i], [0.021667480546618104+1.000266789369622i, -0.00013059902088087365+0.0001035530813307493i, 1.0+0.0i, 1.0+0.0i], [0.0436607778564319+1.0001804866206725i, -8.735516738020677e-05+3.889576665191044e-05i, 1.0+0.0i, 1.0+0.0i], [0.06449697829003033+1.000408654667916i, -3.166249611321768e-05-1.3981660909205915e-05i, 1.0+0.0i, 1.0+0.0i], [0.08391317799483462+0.998837524628444i, 2.4538463509062388e-05-7.002277693063898e-05i, 1.0+0.0i, 1.0+0.0i], [0.10290015988334145+0.9975167601003165i, 5.1350063085285844e-05-0.000112558866692047i, 1.0+0.0i, 1.0+0.0i], [0.120539997651031+0.9956299125744695i, 9.4619136097124e-05-0.000173838122966134i, 1.0+0.0i, 1.0+0.0i], [0.13920193906813186+0.9941959892829693i, 0.0001203264762262389-0.00022050148696545479i, 1.0+0.0i, 1.0+0.0i], [0.1568513205517108+0.9925996183617041i, 0.00014239834438493513-0.0002516640344538403i, 1.0+0.0i, 1.0+0.0i], [0.17287914071443053+0.9895330779397599i, 0.00016188284333777032-0.0003009267007294305i, 1.0+0.0i, 1.0+0.0i], [0.1890063122288304+0.9866353988688106i, 0.00018253999470336114-0.00033447110554740803i, 1.0+0.0i, 1.0+0.0i], [0.2044750517194822+0.9841078596011466i, 0.00018939745929568203-0.00036216968232861437i, 1.0+0.0i, 1.0+0.0i], [0.21954033343846294+0.9813672362472897i, 0.00020876394235480226-0.0004043070209509638i, 1.0+0.0i, 1.0+0.0i], [0.23404455123990153+0.978276961350826i, 0.0002134562818777782-0.00042377395776054786i, 1.0+0.0i, 1.0+0.0i], [0.2475301010835804+0.975030136045388i, 0.00022270630225607537-0.000450207344856095i, 1.0+0.0i, 1.0+0.0i], [0.2619186237351548+0.9715063514728688i, 0.00022316538009615808-0.000480434655781008i, 1.0+0.0i, 1.0+0.0i], [0.2756080302770208+0.9688745834681342i, 0.00021984820443850969-0.0005120357743071701i, 1.0+0.0i, 1.0+0.0i], [0.2879017480329305+0.9650648951131723i, 0.0002136718436752065-0.0005183877471809132i, 1.0+0.0i, 1.0+0.0i], [0.3004358927288185+0.9615177353591898i, 0.00022459620372748584-0.0005379598990331549i, 1.0+0.0i, 1.0+0.0i], [0.31184907036604204+0.9577656755285254i, 0.00021500639188683807-0.0005514566220347263i, 1.0+0.0i, 1.0+0.0i], [0.3243425458435843+0.9537898904013796i, 0.00020096588164041201-0.0005545170337756871i, 1.0+0.0i, 1.0+0.0i], [0.3361774899789625+0.9509079584957769i, 0.00020395073769725533-0.000575795073212864i, 1.0+0.0i, 1.0+0.0i], [0.346726663018472+0.9467741220941969i, 0.00020398361688205198-0.0005802923139815764i, 1.0+0.0i, 1.0+0.0i], [0.3574746962995875+0.9430241278669331i, 0.00018993428592767973-0.0005787913028376093i, 1.0+0.0i, 1.0+0.0i], [0.36740541060046156+0.9391786358686159i, 0.00017675313681701416-0.000602084712863067i, 1.0+0.0i, 1.0+0.0i], [0.37820939645369633+0.934992582608047i, 0.00017868856599528594-0.000595246318497784i, 1.0+0.0i, 1.0+0.0i], [0.38865262531367895+0.9319371825243942i, 0.00017420467735049404-0.0005969810836262253i, 1.0+0.0i, 1.0+0.0i], [0.3976914621938126+0.9276212225312879i, 0.00016660632129207337-0.0005964322360113907i, 1.0+0.0i, 1.0+0.0i], [0.40716348735380564+0.9233936600973643i, 0.00015237337928756248-0.0005971862057168838i, 1.0+0.0i, 1.0+0.0i], [0.4157167896689437+0.9197029641430617i, 0.00015128031371940462-0.000593039195038662i, 1.0+0.0i, 1.0+0.0i], [0.42511963783575096+0.91575941215343i, 0.00015239864432186405-0.000596773451166974i, 1.0+0.0i, 1.0+0.0i], [0.4343902542476348+0.9123871124494441i, 0.00013514814786436003-0.0005929972753201662i, 1.0+0.0i, 1.0+0.0i], [0.4416876046796669+0.9081174917178121i, 0.00013046594807826777-0.0005894870444303165i, 1.0+0.0i, 1.0+0.0i], [0.45051949157568943+0.9037516164042532i, 0.00012082152320519035-0.0005897948072937735i, 1.0+0.0i, 1.0+0.0i], [0.45923740398578866+0.9006780055059861i, 0.00010847864469773086-0.0005939590339605656i, 1.0+0.0i, 1.0+0.0i], [0.4663857240408784+0.896454527416514i, 0.00010870031033054011-0.0005787091905082934i, 1.0+0.0i, 1.0+0.0i], [0.47416037157380325+0.8924775566510694i, 0.00010073772769550092-0.0005796234870044834i, 1.0+0.0i, 1.0+0.0i], [0.4809737528392698+0.8887576717799934i, 8.823713877346466e-05-0.0005712664736627384i, 1.0+0.0i, 1.0+0.0i], [0.48872931994320107+0.8845710372115925i, 7.944433287447089e-05-0.0005707040029714074i, 1.0+0.0i, 1.0+0.0i], [0.49666303960184816+0.8815064828537078i, 8.377321909680296e-05-0.0005612009943789882i, 1.0+0.0i, 1.0+0.0i], [0.5028516483363704+0.8772153017934323i, 7.980243994084632e-05-0.0005501011799364236i, 1.0+0.0i, 1.0+0.0i], [0.5097043507591191+0.8735020416501594i, 7.40614731446556e-05-0.000537978776531183i, 1.0+0.0i, 1.0+0.0i], [0.5157299002956184+0.869817080510211i, 6.644573944950542e-05-0.0005452516272917617i, 1.0+0.0i, 1.0+0.0i], [0.5226497785183872+0.8655127208106937i, 6.135446526078535e-05-0.0005369397710581284i, 1.0+0.0i, 1.0+0.0i], [0.5298204264255573+0.862539272941718i, 5.414088156719705e-05-0.0005203370224305134i, 1.0+0.0i, 1.0+0.0i], [0.5352659401875803+0.858520557927726i, 4.687957616296618e-05-0.0005113022400090897i, 1.0+0.0i, 1.0+0.0i], [0.5413241047463369+0.8548184302035955i, 4.7071745006896605e-05-0.0005042506094732092i, 1.0+0.0i, 1.0+0.0i], [0.5468744328588191+0.8513139342085229i, 4.6625481106394674e-05-0.0004927091212423014i, 1.0+0.0i, 1.0+0.0i], [0.5530709835916716+0.8474663952415775i, 2.8204888301784773e-05-0.0004915727538563128i, 1.0+0.0i, 1.0+0.0i], [0.5593438724313131+0.8443359498126894i, 3.0099897457442164e-05-0.0004858291547648531i, 1.0+0.0i, 1.0+0.0i], [0.5636421777538095+0.8405523453306376i, 2.8465783451510836e-05-0.0004785988885638653i, 1.0+0.0i, 1.0+0.0i], [0.5695840631224391+0.8363228240417405i, 2.1941565387790566e-05-0.00046356063738563983i, 1.0+0.0i, 1.0+0.0i], [0.5757341825438773+0.8336515355503001i, 1.978610727287039e-05-0.00046285829952390326i, 1.0+0.0i, 1.0+0.0i], [0.5803233432042363+0.829548220533113i, 1.044555816815965e-05-0.0004541273368228912i, 1.0+0.0i, 1.0+0.0i], [0.585334470762269+0.8261054967850616i, 5.270037116992032e-06-0.0004429301685563958i, 1.0+0.0i, 1.0+0.0i], [0.5898836066461255+0.8227939331165136i, 9.169669406218192e-06-0.0004363079321682358i, 1.0+0.0i, 1.0+0.0i], [0.5950186700904122+0.8188046336227056i, 3.827167864186326e-06-0.00042852205614610277i, 1.0+0.0i, 1.0+0.0i], [0.6008456414615545+0.8161821879996144i, 5.9927466173177435e-06-0.00042787647387101496i, 1.0+0.0i, 1.0+0.0i], [0.6048288668787071+0.812487638157956i, -6.335591047861467e-06-0.0004154880287120482i, 1.0+0.0i, 1.0+0.0i], [0.609337185323164+0.8089890207489698i, -4.952287241612718e-06-0.0004065498277873962i, 1.0+0.0i, 1.0+0.0i], [0.6134129406981605+0.8057620832938305i, -2.340732610648628e-05-0.00039740282965957996i, 1.0+0.0i, 1.0+0.0i], [0.6181892458883356+0.801960869478003i, -9.86929146982987e-06-0.00039934284970106717i, 1.0+0.0i, 1.0+0.0i], [0.6234142224968502+0.7994403417012501i, -1.312136834937612e-05-0.000384769037638771i, 1.0+0.0i, 1.0+0.0i], [0.6269116004981798+0.795869929984542i, -6.917037154568711e-06-0.0003791143523274684i, 1.0+0.0i, 1.0+0.0i], [0.6311575523088607+0.7926309397134211i, -1.5261703772541134e-05-0.00037345360234701763i, 1.0+0.0i, 1.0+0.0i], [0.634762313985432+0.789517263278661i, -1.998483408662612e-05-0.00036568100845828363i, 1.0+0.0i, 1.0+0.0i], [0.6390256744078681+0.7857964919549795i, -1.9642300777704452e-05-0.0003614207385762048i, 1.0+0.0i, 1.0+0.0i], [0.64392327675904+0.7833779471297915i, -2.01503725962011e-05-0.0003543676029389078i, 1.0+0.0i, 1.0+0.0i], [0.6471512270848832+0.7799285701862104i, -1.786987705149122e-05-0.0003496992544859934i, 1.0+0.0i, 1.0+0.0i], [0.6510198061305829+0.7769054359491976i, -1.4096009284111388e-05-0.0003484077819717761i, 1.0+0.0i, 1.0+0.0i], [0.654394727195776+0.7739109075303251i, -2.1834509901621236e-05-0.0003303245101131376i, 1.0+0.0i, 1.0+0.0i], [0.6584176895238505+0.7706571850086631i, -2.3499287458072333e-05-0.0003273344727761668i, 1.0+0.0i, 1.0+0.0i], [0.6619481986168326+0.7676124110723046i, -2.7693782675722312e-05-0.00032019248313213674i, 1.0+0.0i, 1.0+0.0i], [0.66519600876411+0.7647798667162015i, -1.7528504545714967e-05-0.0003277379592811264i, 1.0+0.0i, 1.0+0.0i], [0.6686825761594151+0.7611957750427011i, -3.206477856160387e-05-0.00031171729133940175i, 1.0+0.0i, 1.0+0.0i], [0.6733543007076233+0.7590018693773981i, -3.729579869036644e-05-0.00030596142074583953i, 1.0+0.0i, 1.0+0.0i], [0.6759126516718741+0.7556584120431196i, -3.2658828396086616e-05-0.00028850011933430374i, 1.0+0.0i, 1.0+0.0i], [0.6791233113270518+0.7528515192210012i, -2.5058147671370256e-05-0.0002853970156157718i, 1.0+0.0i, 1.0+0.0i], [0.6820529972586763+0.7500993889718951i, -4.041445047779588e-05-0.00028785939640703324i, 1.0+0.0i, 1.0+0.0i], [0.6853987524868371+0.7465498560154481i, -3.2516063744737426e-05-0.0002844711838476917i, 1.0+0.0i, 1.0+0.0i], [0.6895717347786313+0.7445573786591395i, -2.757828158665228e-05-0.00027369278834157157i, 1.0+0.0i, 1.0+0.0i], [0.6919096554165745+0.7414559284167299i, -2.978537830561615e-05-0.00026482243712939757i, 1.0+0.0i, 1.0+0.0i]]}  # Simulated Filter Data
  # "Display Units don't matter\nhere since this is not where\nwe create the display traces.\nWe just need to get P/F status."
  n1 = Unbundle By Name("Test Parameters") -> ("Stimulus.Sweep.Units"=w14:T4, "Display.Formatted Data"=w23:bool, "Measurement.Auto Select"=w33:bool, "Filter Limits"=w11:T35[], "Limits"=w2:T31[], "Measurement.Parameters"=w38:T23[], "Stimulus.Calibration"=w34:T11, "Stimulus"=w37:T21, "Measurement.Data Source"=w31:enum16{"VNA", "Data File"}, "De-Embed.De-Embed"=w24:bool, "De-Embed.Adapters"=w25:T25[])
  n2 = case shown="\"Data File\"" w31 {
    tunnel: "error in (no error)" -> [w59 w127]
    tunnel: [w58 w112] -> w28
    tunnel: [w54 w126] -> w5
    tunnel: [w53 w125] -> w17
    tunnel: w38 -> [w71 _]
    tunnel: w37 -> [w56 _]
    tunnel: [w64 w124] -> w36
    tunnel: w34 -> [w69 _]
    tunnel: w23 -> [w67 _]
    tunnel: w33 -> [w66 _]
    tunnel: "Driver Refs" -> [w50 w123]
    tunnel: cluster{"Limits":T31[]}[] [] -> [w63 w116]
    tunnel: w2 -> [w65 w114]
    tunnel: "Timing Metrics In" -> [w61 w111]
    tunnel: [w62 w110] -> w20
    tunnel: "Seq Count" -> [w60 _]
    tunnel: "Instrument Record" -> [w52 _]
    frame "VNA", Default {
      # "Normal VNA interaction."
      n3 = Bundle By Name(cluster=T45 {"Formatted Data"=FALSE, "Auto Select"=FALSE, "Seq Count"=0} ("Miscellaneous Parameters"), "Seq Count"=w60, "Formatted Data"=w67, "Auto Select"=w66) -> (w57:T45)
      n4 = Unbundle By Name(w52) -> ("sDriverType"=w51:string)
      n5 = for {
        tunnel: w71 -> [w106] mode=indexing
        tunnel: [w105] -> w55 mode=indexing
        tunnel: w69 -> [w104]
        tunnel: T10 {"Channel"=0, "Parameter"={"Stimulus Port"=0, "Response Port"=0}, "Calibration"={"State"=FALSE, "String"=""}, "Display Format"=enum."Log Mag", "Pass?"=FALSE} ("Parameter to Measure") -> [w103]
        tunnel: w65 -> [w101]
        shift-right: [w97] -> w64
        shift-left: w63 -> [w98]
        n6 = Unbundle By Name(w106) -> ("Channel"=w102:i8, "Parameter"=w100:T2)
        n7 = call "SP Find Limit by Parameter.vi"("Parameter"=w100, "Limits"=w101) -> ("Limits"=w99:T31[])  [unwired: 9 out]
        n8 = Bundle("Limits"=w99) -> (w96:cluster{"Limits":T31[]})  [unwired: 1 in]
        n9 = Build Array (concatenate)(w98, w96) -> (w97:cluster{"Limits":T31[]}[])
        n10 = Bundle(cluster=w103, "Channel"=w102, "Parameter"=w100, "Calibration"=w104) -> (w105:T10)  [unwired: 2 out]
      }
      n11 = case shown="\"VNA\", Default" w51 {
        tunnel: w59 -> [w81 w91]
        tunnel: w57 -> [w80 w90]
        tunnel: w55 -> [w79 w89]
        tunnel: [w78 w88] -> w58
        tunnel: w56 -> [w76 w86]
        tunnel: [w74 w84] -> w54
        tunnel: [w75 w85] -> w53
        tunnel: w50 -> [w73 w83]
        frame "VNA", Default {
          n12 = Unbundle By Name(w73) -> ("VNA Driver Ref"=w72:T17)
          n13 = call "VNA Driver.vi"("Drv Refnum"=w72, "VNA Command"=VNA_Command."MEASURE", "error in (no error)"=w81, "Miscellaneous Parameters"=w80, "VNA Stimulus"=w76, "Parameters to Measure"=w79) -> ("error out"=w78:errorcluster, "SP Data"=w74:T26, "Parameters Measured"=w75:T10[])  [unwired: 1 in, 2 out]
        }
        frame "SNA" {
          n14 = Unbundle By Name(w83) -> ("SNA Driver Ref"=w82:T18)
          n15 = call "SNA Driver.vi"("Drv Refnum"=w82, "SNA Command"=SNA_Command."MEASURE", "error in (no error)"=w91, "Miscellaneous Parameters"=w90, "SNA Stimulus"=w86, "Parameters to Measure"=w89) -> ("error out"=w88:errorcluster, "SP Data"=w84:T26, "Parameters Measured"=w85:T10[])  [unwired: 1 in, 2 out]
        }
      }
      n16 = stacked-sequence {
        tunnel: [w95] -> w62
        tunnel: w61 -> [w92]
        tunnel: w58 -> [_]
        frame #0 {
          n17 = call "Test Timing Metrics.vi"("Start?"=FALSE, "Timing Metrics In"=w92, "Message"="Driver Measurements Completed: NA") -> ("Timing Metrics Out"=w95:string)  [unwired: 6 out]
        }
      }
    }
    frame "Data File" {
      w113 = 4
      # "Format the limits so they can still be applied to imported data.  They must be in the order of S11, S21, S12, S22 because that is the order that S2P data comes back from the driver.  This is not a requirement of ours, but rather the requirement of the Touchstone (S2P) format.  If there is not a limit for that SP it needs to have a blank entry to fulfill the requirements of the code to come. - CHB"
      n18 = Unbundle By Name(w123) -> ("IMP Driver Ref"=w121:T19)
      n19 = Index Array(array=w116) -> (element=w115:cluster{"Limits":T31[]})  [unwired: 1 in]
      n20 = Initialize Array(w115, w113) -> (w117:cluster{"Limits":T31[]}[])
      n21 = call "IMP Driver.vi"("Drv Refnum"=w121, "IMP Command"=IMP_Command."IMPORT" ("VNA Command"), "error in (no error)"=w127) -> ("error out"=w108:errorcluster, "Variant Output"=w119:variant)  [unwired: 2 in, 5 out]
      n22 = Unbundle(w108) -> ("code"=w109:i32)  [unwired: 2 out]
      n23 = for {
        N: w113 -> [_]
        shift-right: [w138] -> w124
        shift-left: w117 -> [w139]
        tunnel: w114 -> [w134]
        i -> [w136]
        n24 = case shown="0, Default" w136 {
          tunnel: [T2 {"Stimulus Port"=1, "Response Port"=1} ("Parameter") T2 {"Stimulus Port"=1, "Response Port"=2} ("Parameter") T2 {"Stimulus Port"=2, "Response Port"=1} ("Parameter") T2 {"Stimulus Port"=2, "Response Port"=2} ("Parameter")] -> w135
          frame 0, Default {
          }
          frame 1 {
          }
          frame 2 {
          }
          frame 3 {
          }
        }
        n25 = call "SP Find Limit by Parameter.vi"("Parameter"=w135, "Limits"=w134) -> ("Limits"=w133:T31[])  [unwired: 9 out]
        n26 = Bundle("Limits"=w133) -> (w137:cluster{"Limits":T31[]})  [unwired: 1 in]
        n27 = Replace Array Subset(array=w139, new element=w137, index=w136) -> (w138:cluster{"Limits":T31[]}[])
      }
      n28 = case shown="43" w109 {
        tunnel: w108 -> [w128 _]
        tunnel: [w128 _] -> w107
        frame Default {
        }
        frame 43 {
          # "Clear the error that is\ngenerated when the user\ncnacels.  This will allow the\nuser to click Measure again\nif they choose.  All other\nbutton functions will work\nas well, i.e. Abort, Abort All, \netc."
        }
      }
      n29 = Variant To Data(error in=w107, type=T48 {"Parameters Measured"=[], "S2P Data"={"F0"=0.0, "dF"=0.0, "Data"=[]}} ("S2P Measurements"), Variant=w119) -> (data=w118:T48, error out=w112:errorcluster)
      n30 = stacked-sequence {
        tunnel: [w132] -> w110
        tunnel: w111 -> [w129]
        tunnel: w112 -> [_]
        frame #0 {
          n31 = call "Test Timing Metrics.vi"("Start?"=FALSE, "Timing Metrics In"=w129, "Message"="Driver Measurements Completed: IMP") -> ("Timing Metrics Out"=w132:string)  [unwired: 6 out]
        }
      }
      n32 = Unbundle By Name(w118) -> ("Parameters Measured"=w125:T10[], "S2P Data"=w126:T26)
    }
  }
  n33 = call "DEBUG.vi"("Dev DEBUG? (f)"=w9) -> ("DEBUG?"=w8:bool)  [unwired: 1 in, 5 out]
  n34 = Not(x=w8) -> (.not. x?=w7:bool)
  n35 = Select(t=w5, s=w7, f=w6) -> (s? t:f=w4:T26)
  n36 = Bundle By Name(cluster=T44 {"Measurement Units"=enum."Hz", "Display Units"=enum."Hz"} ("Units"), "Measurement Units"=w14) -> (w13:T44)
  n37 = call "SP Strip Channel From Parameters.vi"("Parameters to Measure"=w17) -> ("Parameters to Measure"=w27:T2[])  [unwired: 4 out]
  n38 = case shown="False" w24 {
    tunnel: [w144 w151] -> w29
    tunnel: w28 -> [w144 w150]
    tunnel: w27 -> [_ w149]
    tunnel: w4 -> [w145 w148]
    tunnel: [w145 w147] -> w26
    tunnel: w25 -> [_ w146]
    frame False {
    }
    frame True {
      n39 = call "SP De-Embed SP.vi"("error in (no error)"=w150, "Adapters"=w146, "SP Array"=w148, "Measured Parameters"=w149) -> ("error out"=w151:errorcluster, "De-embedded SP Array"=w147:T26)  [unwired: 6 out]
    }
  }
  n40 = Array Size(array=w27) -> (size(s)=w44:i32)
  n41 = Unbundle(w26) -> ("F0"=w42:dbl, "dF"=w41:dbl, "Data"=w40:cdb[][])
  n42 = Index Array(array=w3) -> (element=w1:T1)  [unwired: 1 in]
  n43 = for "For each S parameter measured..." {
    shift-right: [w187] -> w48
    shift-left: w29 -> [w182]
    tunnel: w36 -> [w188] mode=indexing
    tunnel: w27 -> [w164] mode=indexing
    shift-right: [w178] -> w47
    shift-left: "Empty Results" -> [w183]
    tunnel: [w158] -> w19 mode=indexing
    tunnel: w44 -> [w175]
    tunnel: "CH Controls" -> [w173]
    tunnel: w42 -> [w172]
    tunnel: w41 -> [w171]
    tunnel: w40 -> [w170]
    tunnel: [w166] -> w39 mode=indexing
    tunnel: w25 -> [w160]
    tunnel: w13 -> [w159]
    tunnel: w17 -> [w155] mode=indexing
    tunnel: [w157] -> w16 mode=indexing
    tunnel: w11 -> [w156]
    shift-right: [w154] -> w10
    shift-left: w3 -> [w153]
    tunnel: w1 -> [w152]
    i -> [w174]
    # "This picks\nmeasurement\ncolumns ... eg\nS11 mag,\nS11 phase,..."
    n44 = Unbundle(w188) -> ("Limits"=w176:T31[])
    n45 = Index Array(array=w170, index (col)=w174) -> (element=w168:cdb[])  [unwired: 1 in]
    n46 = Equal To 0?(x=w174) -> (x = 0?=w186:bool)
    n47 = Array Size(array=w168) -> (size(s)=w167:i32)
    n48 = case shown="True" w186 {
      tunnel: w168 -> [w374 w384]
      tunnel: [w374 w384] -> w169
      tunnel: w172 -> [w373 w386]
      tunnel: w171 -> [w372 w385]
      tunnel: [w373 w386] -> w185
      tunnel: [w372 w385] -> w184
      tunnel: w183 -> [w371 w388]
      tunnel: w182 -> [w370 w387]
      tunnel: [w370 w377] -> w179
      tunnel: [w371 w378] -> w181
      tunnel: "NI_ChannelName" -> [w369 w381]
      tunnel: [w369 w380] -> w165
      tunnel: w167 -> [_ w383]
      tunnel: w160 -> [_ w375]
      frame False {
      }
      frame True {
        n49 = call "SP Append Frequency Waveform.vi"("Number of Points"=w383, "Attribute Name (NI_ChannelName)"=w381, "error in (no error)"=w387, "dF"=w385, "F0"=w386, "Waveforms in"=w388) -> ("error out"=w376:errorcluster, "Waveforms out"=w379:waveform(dbl)[])  [unwired: 4 out]
        n50 = Array Size(array=w375) -> (size(s)=w382:i32)
        n51 = case shown="Default" w382 {
          tunnel: w381 -> [w391 w393]
          tunnel: [w391 w393] -> w380
          tunnel: w379 -> [w390 w397]
          tunnel: [w390 w396] -> w378
          tunnel: [w389 w394] -> w377
          tunnel: w376 -> [w389 w395]
          tunnel: w375 -> [_ w392]
          frame 0 {
          }
          frame Default {
            n52 = call "SP Append Adapter Waveforms.vi"("Attribute Name (NI_ChannelName)"=w393, "error in (no error)"=w395, "Adapters"=w392, "Waveforms in"=w397) -> ("error out"=w394:errorcluster, "Waveforms out"=w396:waveform(dbl)[])  [unwired: 6 out]
          }
        }
      }
    }
    n53 = call "SP Append Measured Waveform.vi"("Waveforms in"=w181, "Attribute Name (NI_ChannelName)"=w165, "CH Controls"=w173, "Measured Data"=w169, "All Measured Data"=w170, "Current Index"=w174, "error in (no error)"=w179, "Number of Parameters Measured"=w175, "Measured Parameter"=w164) -> ("Waveforms out"=w163:waveform(dbl)[], "Memory Exists?"=w166:bool, "Stored Data"=w162:cdb[], "error out"=w161:errorcluster)  [unwired: 2 in, 1 out]
    n54 = Array Size(array=w176) -> (size(s)=w177:i32)
    n55 = case shown="Default" w177 {
      tunnel: w176 -> [_ w210]
      tunnel: [w191 w209] -> w187
      tunnel: w185 -> [_ w208]
      tunnel: w184 -> [_ w207]
      tunnel: w161 -> [w191 w206]
      tunnel: w163 -> [w192 w205]
      tunnel: [w192 w204] -> w178
      tunnel: w165 -> [_ w203]
      tunnel: w162 -> [_ w202]
      tunnel: w164 -> [_ w201]
      tunnel: [TRUE w197] -> w158
      tunnel: w167 -> [_ w199]
      tunnel: w159 -> [_ w198]
      tunnel: w156 -> [_ w196]
      tunnel: [w190 w195] -> w154
      tunnel: w153 -> [w190 w194]
      tunnel: w152 -> [_ w193]
      frame 0 {
      }
      frame Default {
        n56 = for "For each limit specified...(e.g., both mag and phase limits for an S-parameter)" {
          tunnel: w210 -> [w227] mode=indexing
          shift-right: [w236] -> w209
          shift-left: w206 -> [w232]
          tunnel: w208 -> [w225]
          tunnel: w207 -> [w224]
          shift-right: [w235] -> w204
          shift-left: w205 -> [w234]
          tunnel: w201 -> [w217]
          tunnel: w203 -> [w233]
          tunnel: w202 -> [w223]
          tunnel: [w211] -> w200 mode=indexing
          tunnel: w199 -> [w231]
          tunnel: w198 -> [w230]
          tunnel: w196 -> [w228]
          shift-right: [w214] -> w195
          shift-left: w194 -> [w221]
          tunnel: w193 -> [w219]
          n57 = Unbundle By Name(w227) -> ("Limit Type"=w229:T32, "Limit #"=w216:i8, "Format"=w220:T6)
          n58 = call "SP Format Fundamental Value for Display (complex array).vi"("dF, MHz"=w224, "Sxx Measured Format"=w220, "Fundamental Values"=w223) -> ("Formatted Values"=w226:dbl[])  [unwired: 1 in, 7 out]
          n59 = Bundle By Name(cluster=w219, "Limit #"=w216, "Parameter"=w217) -> (w218:T1)
          n60 = Bundle("F0"=w225, "dF"=w224, "Formatted Values"=w226) -> (w222:T50)  [unwired: 1 out]
          n61 = case shown="\"Filter\"" w229 {
            tunnel: [w247 w342] -> w236
            tunnel: [w252 w341] -> w235
            tunnel: w217 -> [w245 w340]
            tunnel: [w254 w323] -> w211
            tunnel: w234 -> [w253 w321]
            tunnel: w233 -> [w243 w319]
            tunnel: w232 -> [w248 w317]
            tunnel: w224 -> [_ w302]
            tunnel: w225 -> [_ w303]
            tunnel: w231 -> [w242 w307]
            tunnel: w230 -> [_ w306]
            tunnel: w228 -> [w251 _]
            tunnel: w227 -> [_ w305]
            tunnel: w220 -> [w244 w304]
            tunnel: [w246 w300] -> w215
            tunnel: w222 -> [w241 w301]
            tunnel: w221 -> [w240 w300]
            tunnel: w216 -> [w239 _]
            tunnel: w218 -> [w238 w299]
            tunnel: [w237 w299] -> w212
            frame "Filter" {
              n62 = call "SP Find Filter Limit by Limit #.vi"("Limit #"=w239, "Filter Limits"=w251) -> ("Found?"=w250:bool, "Filter Limit"=w249:T35)  [unwired: 8 out]
              n63 = case shown="True" w250 {
                tunnel: [w286 TRUE] -> w254
                tunnel: w253 -> [w293 w298]
                tunnel: [w292 w298] -> w252
                tunnel: w249 -> [w289 _]
                tunnel: w248 -> [w291 w297]
                tunnel: [w290 w297] -> w247
                tunnel: w241 -> [w288 _]
                tunnel: [w255 w295] -> w246
                tunnel: w245 -> [w285 _]
                tunnel: w244 -> [w284 _]
                tunnel: w243 -> [w283 _]
                tunnel: w242 -> [w282 _]
                tunnel: w240 -> [w255 w295]
                tunnel: w238 -> [w257 w294]
                tunnel: [w256 w294] -> w237
                frame True {
                  n64 = Unbundle By Name(w289) -> ("Filter Type"=w258:T36)
                  n65 = call "SP Perform Filter Bandwidth Limit Testing.vi"("Limit Results In"=w257, "error in (no error)"=w291, "Data"=w288, "Filter Limit"=w289) -> ("error out"=w267:errorcluster, "Results"=w265:T51, "Pass?"=w259:bool, "Limit Results Out"=w280:T1)  [unwired: 4 out]
                  n66 = call "SP Append Filter Bandwidth Limit Waveform.vi"("Limit Format"=w284, "Measured Parameter"=w285, "Attribute Name (NI_ChannelName)"=w283, "error in (no error)"=w267, "Filter Type"=w258, "Results"=w265, "Waveforms in"=w293) -> ("error out"=w266:errorcluster, "Waveforms out"=w268:waveform(dbl)[])  [unwired: 1 in, 2 out]
                  n67 = call "SP Perform Filter Ripple Limit Testing.vi"("Filter Limit"=w289, "Data"=w288, "error in (no error)"=w266, "Limit Results In"=w280) -> ("Limits Pass/Fail"=w276:cluster{"Upper Pass?":bool, "Lower Pass?":bool}, "Upper and Lower Limits"=w275:T52, "Limit Results Out"=w279:T1, "error out"=w273:errorcluster)  [unwired: 2 in, 6 out]
                  n68 = Cluster To Array(cluster=w276) -> (array=w277:bool[])
                  n69 = call "SP Append Filter Ripple Limit Waveform.vi"("Limit Format"=w284, "Number of Points"=w282, "Measured Parameter"=w285, "Attribute Name (NI_ChannelName)"=w283, "error in (no error)"=w273, "Limits Pass/Fail"=w276, "Upper and Lower Limits"=w275, "Waveforms in"=w268) -> ("error out"=w272:errorcluster, "Waveforms out"=w264:waveform(dbl)[])  [unwired: 2 out]
                  n70 = call "SP Perform Filter Attenuation Limit Testing.vi"("Limit Results In"=w279, "error in (no error)"=w272, "Data"=w288, "Filter Limit"=w289) -> ("error out"=w262:errorcluster, "Results"=w260:T53, "Pass?"=w281:bool, "Limit Results Out"=w278:T1)  [unwired: 4 out]
                  n71 = call "SP Append Filter Attenuation Limit Waveform.vi"("Limit Format"=w284, "Measured Parameter"=w285, "Attribute Name (NI_ChannelName)"=w283, "error in (no error)"=w262, "Results"=w260, "Waveforms in"=w264) -> ("error out"=w261:errorcluster, "Waveforms out"=w263:waveform(dbl)[])  [unwired: 4 out]
                  n72 = call "SP Perform Filter Skirt Limit Testing.vi"("Filter Limit"=w289, "Data"=w288, "error in (no error)"=w261, "Limit Results In"=w278) -> ("Limits Pass/Fail"=w270:cluster{"Upper Pass?":bool, "Lower Pass?":bool}, "Upper and Lower Limits"=w269:T52, "Limit Results Out"=w256:T1, "error out"=w271:errorcluster)  [unwired: 2 in, 6 out]
                  n73 = Cluster To Array(cluster=w270) -> (array=w274:bool[])
                  n74 = call "SP Append Filter Skirt Limit Waveform.vi"("Limit Format"=w284, "Number of Points"=w282, "Measured Parameter"=w285, "Attribute Name (NI_ChannelName)"=w283, "error in (no error)"=w271, "Limits Pass/Fail"=w270, "Upper and Lower Limits"=w269, "Waveforms in"=w263) -> ("error out"=w290:errorcluster, "Waveforms out"=w292:waveform(dbl)[])  [unwired: 2 out]
                  n75 = Compound Arithmetic op=AND(w274, w281, w277, w259) -> (w287:bool[])
                  n76 = And Array Elements(Boolean array=w287) -> (logical AND=w286:bool)
                }
                frame False {
                }
              }
            }
            frame "Upper".."Delta", "Referential" {
              # "We have to perform the limit testing here, so\nwe test all of the requirements, not just those\nthe user has chosen to view..."
              # "Limits are created here and saved in there own waveforms...Note that we\ndo the Limit Creation in the units in which the user specified the limit,\nthen we transform back to base units for the storage..."
              # "We have to and the trues together\nafter the loop so that we do not\nhave to worry about how many\ntimes the loop has been run."
              n77 = Build Array(w305) -> (w316:T31[])
              n78 = call "SP Coerce Limts to Valid Values.vi"("Attribute Name (NI_ChannelName)"=w319, "error in (no error)"=w317, "Units"=w306, "Limits"=w316, "Results"=w321) -> ("error out"=w310:errorcluster, "Lower Limit Traces"=w311:cluster{"X":dbl[], "Y":dbl[]}[], "Upper Limit Traces"=w318:cluster{"X":dbl[], "Y":dbl[]}[], "dup Results"=w320:waveform(dbl)[])  [unwired: 3 out]
              n79 = Array Size(array=w318) -> (size(s)=w343:i32)
              n80 = Array Size(array=w311) -> (size(s)=w312:i32)
              n81 = case shown="1.." w312 {
                tunnel: [w347 w356] -> w309
                tunnel: w310 -> [w349 w355]
                tunnel: [w349 w354] -> w308
                tunnel: w303 -> [w346 w353]
                tunnel: w302 -> [w345 w352]
                tunnel: w311 -> [_ w351]
                frame 0, Default {
                  n82 = Bundle(cluster=cluster{"x0":dbl, "dx":dbl, "Y":dbl[]} {"x0"=0.0, "dx"=0.0, "Y"=[]} ("Limit"), "x0"=w346, "dx"=w345) -> (w347:cluster{"x0":dbl, "dx":dbl, "Y":dbl[]})  [unwired: 1 out]
                }
                frame 1.. {
                  n83 = call "SP Create Segmented Mask.vi"("Reset"=TRUE, "error in"=w355, "x0"=w353, "dx"=w352, "Specification Cluster"=w351) -> ("error out"=w354:errorcluster, "Limit"=w356:cluster{"x0":dbl, "dx":dbl, "Y":dbl[]})  [unwired: 3 out]
                }
              }
              n84 = case shown="1.." w343 {
                tunnel: [w359 w368] -> w313
                tunnel: w310 -> [w361 w367]
                tunnel: [w361 w366] -> w344
                tunnel: w303 -> [w358 w365]
                tunnel: w302 -> [w357 w364]
                tunnel: w318 -> [_ w363]
                frame 0, Default {
                  n85 = Bundle(cluster=cluster{"x0":dbl, "dx":dbl, "Y":dbl[]} {"x0"=0.0, "dx"=0.0, "Y"=[]} ("Limit"), "x0"=w358, "dx"=w357) -> (w359:cluster{"x0":dbl, "dx":dbl, "Y":dbl[]})  [unwired: 1 out]
                }
                frame 1.. {
                  n86 = call "SP Create Segmented Mask.vi"("Reset"=TRUE, "error in"=w367, "x0"=w365, "dx"=w364, "Specification Cluster"=w363) -> ("error out"=w366:errorcluster, "Limit"=w368:cluster{"x0":dbl, "dx":dbl, "Y":dbl[]})  [unwired: 3 out]
                }
              }
              n87 = Merge Errors(w344, w308) -> (w331:errorcluster)
              n88 = Build Array(w309) -> (w314:cluster{"x0":dbl, "dx":dbl, "Y":dbl[]}[])
              n89 = Build Array(w313) -> (w315:cluster{"x0":dbl, "dx":dbl, "Y":dbl[]}[])
              n90 = Unbundle(w313) -> ("x0"=w339:dbl, "dx"=w338:dbl, "Y"=w337:dbl[])
              n91 = Unbundle(w309) -> ("x0"=w333:dbl, "dx"=w332:dbl, "Y"=w334:dbl[])
              n92 = call "SP Perform Limit Testing.vi"("Generate Plot Output? (f)"=FALSE, "error in (no error)"=w331, "LLimits"=w314, "ULimits"=w315, "Data"=w301) -> ("error out"=w330:errorcluster, "Lower Pass?"=w324:bool, "Upper Pass?"=w325:bool)  [unwired: 2 in, 2 out]
              n93 = call "SP Format Value to Fundamental (array).vi"("Sxx Display Format"=w304, "Display Values"=w337) -> ("Stored Values"=w336:dbl[])  [unwired: 5 out]
              n94 = call "SP Format Value to Fundamental (array).vi"("Sxx Display Format"=w304, "Display Values"=w334) -> ("Stored Values"=w335:dbl[])  [unwired: 5 out]
              n95 = And(x=w325, y=w324) -> (x .and. y?=w323:bool)
              n96 = Bundle("x0"=w339, "dx"=w338, "Stored Values"=w336) -> (w329:T54)  [unwired: 1 out]
              n97 = Bundle("x0"=w333, "dx"=w332, "Stored Values"=w335) -> (w328:T54)  [unwired: 1 out]
              n98 = Bundle("Upper Pass?"=w325, "Lower Pass?"=w324) -> (w326:cluster{"Upper Pass?":bool, "Lower Pass?":bool})  [unwired: 1 out]
              n99 = Bundle(w329, w328) -> (w327:T55)  [unwired: 1 out]
              n100 = call "SP Append Limit Waveform.vi"("Limit Format"=w304, "Number of Points"=w307, "Measured Parameter"=w340, "Attribute Name (NI_ChannelName)"=w319, "error in (no error)"=w330, "Limits Pass/Fail"=w326, "Upper and Lower Limits"=w327, "Waveforms in"=w320) -> ("error out"=w342:errorcluster, "Waveforms out"=w341:waveform(dbl)[])  [unwired: 2 out]
            }
          }
          n101 = Bundle By Name(cluster=w212, "Pass?"=w211) -> (w213:T1)
          n102 = Build Array (concatenate)(w215, w213) -> (w214:T1[])
        }
        n103 = And Array Elements(Boolean array=w200) -> (logical AND=w197:bool)
      }
    }
    n104 = Bundle By Name(cluster=w155, "Pass?"=w158) -> (w157:T10)
  }
  "error out" <- w48
  "Results" <- w47
  "Memory Exists?" <- w39
  "Parameters Measured" <- w16
  "Limit Results" <- w10
  n105 = stacked-sequence {
    tunnel: [w401] -> w21
    tunnel: w20 -> [w398]
    tunnel: w19 -> [_]
    frame #0 {
      n106 = call "Test Timing Metrics.vi"("Start?"=FALSE, "Timing Metrics In"=w398, "Message"="Data Processed") -> ("Timing Metrics Out"=w401:string)  [unwired: 6 out]
    }
  }
  "Timing Metrics Out" <- w21
  n107 = And Array Elements(Boolean array=w19) -> (logical AND=→"Passed?":bool)
